vi "Load Unit Test Paths.vi"(8 "Error In":errorcluster, 9 "Challenge Config File":path, 10 "Challenge Config":T1, 11 "Config File Handle":T2) -> (0 "Error Out":errorcluster, 2 "Challenge Config":T1, 3 "Config File Handle":T2)   [LabVIEW 2013, in "VIChallenge.lvlib"]
doc: "Load unit tests by reading from the challenge config file."
uses:
  VIChallenge.lvlib
  <vilib>/Utility/config.llb/NI_LVConfig.lvlib
  <vilib>/Utility/config.llb/Read Key (Boolean).vi
  <vilib>/Utility/config.llb/Config Data RefNum.ctl
  Type Defs/Challenge.ctl
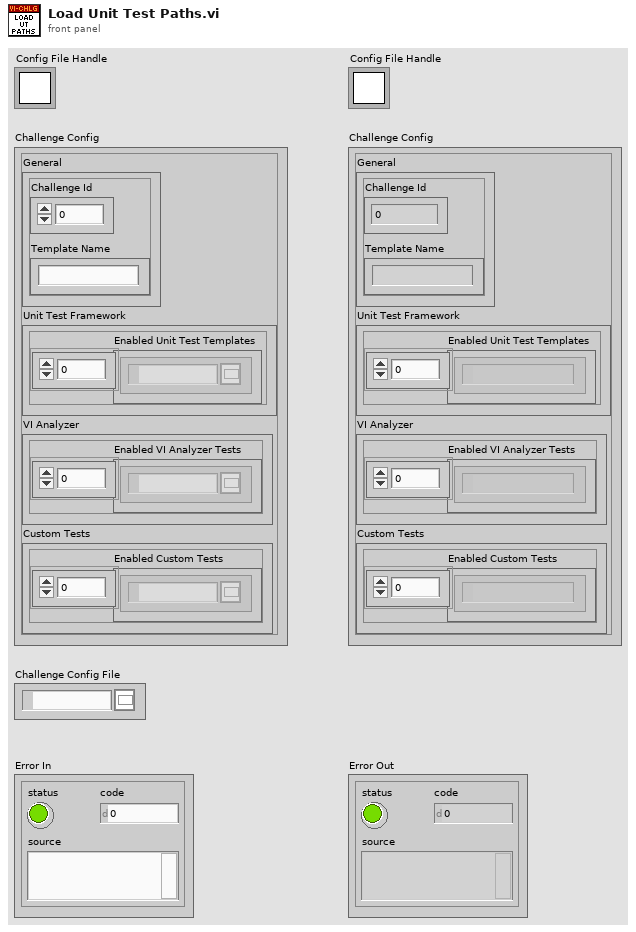
[diagram p1: front panel]
types:
  T1 = typedef "VIChallenge.lvlib/Challenge.ctl" = cluster{"General":cluster{"Challenge Id":i32, "Template Name":string}, "Unit Test Framework":cluster{"Enabled Unit Test Templates":path[]}, "VI Analyzer":cluster{"Enabled VI Analyzer Tests":path[]}, "Custom Tests":cluster{"Enabled Custom Tests":path[]}}
  T2 = typedef "NI_LVConfig.lvlib/Config Data RefNum.ctl" = refnum<k1>
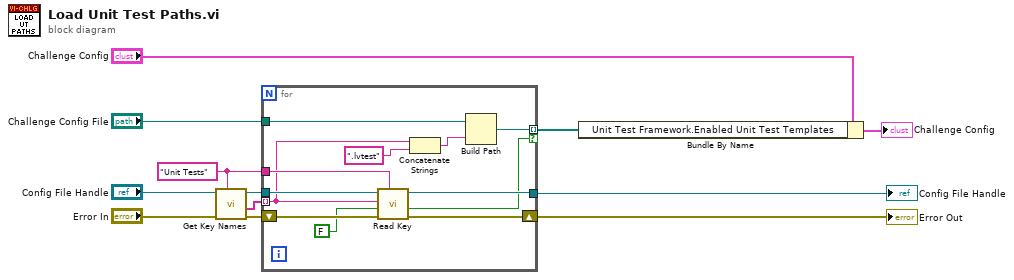
[diagram p0: block diagram]
diagram:
  w9 = "Unit Tests" ("section")
  n1 = call <vilib>:"Get Key Names.vi"("section"=w9, "error in (no error)"="Error In", "refnum"="Config File Handle") -> ("error out"=w6:errorcluster, "key names"=w8:string[], "refnum out"=w7:T2)  [unwired: 5 in, 1 out]
  n2 = for {
    tunnel: w7 -> [w23]
    tunnel: w8 -> [w15] mode=indexing
    tunnel: w9 -> [w21]
    tunnel: [w20] -> w10
    shift-right: [w19] -> w11
    shift-left: w6 -> [w24]
    tunnel: "Challenge Config File" -> [w18]
    tunnel: [w17] -> w1 mode=indexing if=w16
    n3 = call-poly <vilib>:"Read Key.vi"("section"=w21, "error in (no error)"=w24, "default value"=FALSE, "key"=w15, "refnum"=w23) -> ("error out"=w19:errorcluster, "value"=w16:bool, "refnum out"=w20:T2)  [unwired: 3 in, 1 out]
    n4 = Concatenate Strings(w15, ".lvtest" ("string")) -> (w13:string)
    n5 = Build Path(base path=w18, name or relative path=w13) -> (appended path=w17:path)
  }
  "Error Out" <- w11
  "Config File Handle" <- w10
  n6 = Bundle By Name(cluster="Challenge Config", "Unit Test Framework.Enabled Unit Test Templates"=w1) -> (→"Challenge Config":T1)
